vi "Check-client-activity.vi"(8 "error in (no error)":errorcluster, 9 "Check period":u32=5000 caption="Check period [ms]", 11 "ModComm in":T1) -> (0 "error out":errorcluster, 3 "ModComm out":T1)   [LabVIEW 2013, in "Server.lvlib" / "Server.lvclass"]
uses:
  Server.lvclass
  Object-reference.ctl
  Server.lvclass/Server.ctl
  Read Client IDs.vi
  Read Last contact.vi
  Read Heartbeat timeout.vi
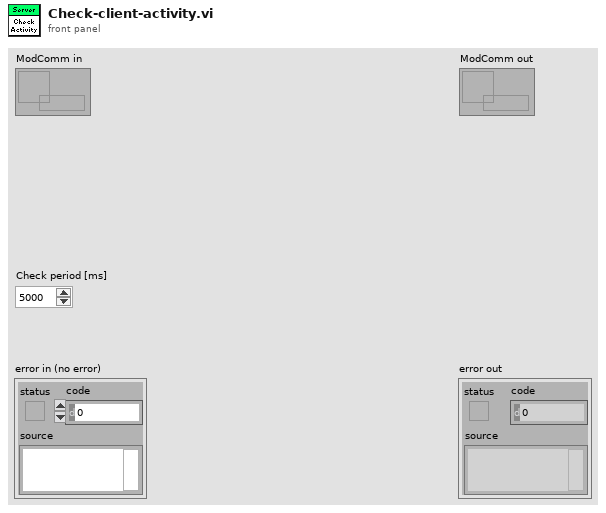
[diagram p1: front panel]
types:
  T1 = typedef "Server.lvlib/Server.lvclass/Object-reference.ctl" = refnum<data-value>
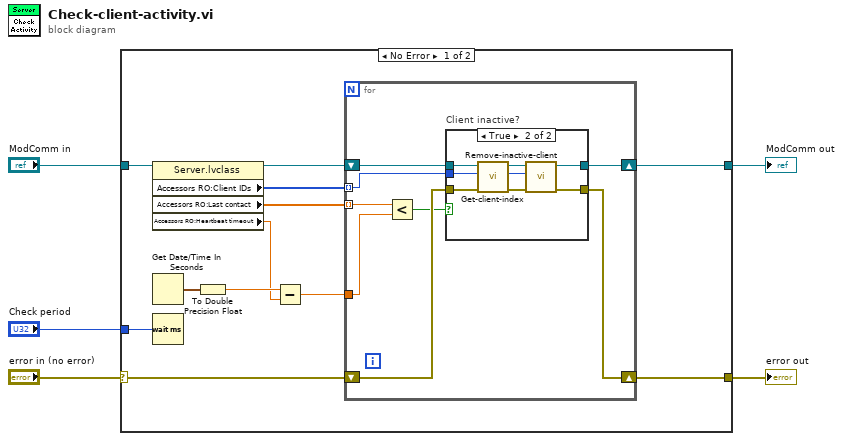
[diagram p0: block diagram]
diagram:
  n1 = case shown="No Error" "error in (no error)" {
    selector: "error in (no error)" -> [w7 w37]
    tunnel: [w6 w37] -> w4
    tunnel: [w8 w36] -> w2
    tunnel: "ModComm in" -> [w17 w36]
    tunnel: "Check period" -> [w16 _]
    frame No Error {
      n2 = property class="Server.lvclass"(reference=w17) -> (reference out=w9:T1, "Accessors RO:Client IDs"=w11:i32[], "Accessors RO:Last contact"=w12:dbl[], "Accessors RO:Heartbeat timeout"=w13:dbl)  [unwired: 1 in, 1 out]
      n3 = Get Date/Time In Seconds() -> (seconds since 1Jan1904=w15:timestamp)
      n4 = Wait (ms)(milliseconds to wait=w16) -> ()  [unwired: 1 out]
      n5 = To Double Precision Float(number=w15) -> (double precision float=w14:dbl)
      n6 = Subtract(x=w14, y=w13) -> (x-y=w10:dbl)
      n7 = for {
        tunnel: w12 -> [w25] mode=indexing
        tunnel: w11 -> [w18] mode=indexing
        tunnel: w10 -> [w24]
        shift-right: [w22] -> w8
        shift-left: w9 -> [w23]
        shift-right: [w20] -> w6
        shift-left: w7 -> [w21]
        n8 = Less?(x=w25, y=w24) -> (x < y?=w19:bool)
        n9 = case "Client inactive?" shown="True" w19 {
          tunnel: w23 -> [w27 w33]
          tunnel: [w27 w35] -> w22
          tunnel: w21 -> [w26 w29]
          tunnel: [w26 w34] -> w20
          tunnel: w18 -> [_ w30]
          frame False {
          }
          frame True {
            n10 = call "Get-client-index.vi"("error in (no error)"=w29, "Client ID"=w30, "ModComm in"=w33) -> ("error out"=w28:errorcluster, "Client index"=w31:i32, "ModComm out"=w32:T1)  [unwired: 6 in]
            n11 = call "Remove-inactive-client.vi"("error in (no error)"=w28, "Client index"=w31, "ModComm in"=w32) -> ("error out"=w34:errorcluster, "ModComm out"=w35:T1)  [unwired: 7 in]
          }
        }
      }
    }
    frame Error {
    }
  }
  "error out" <- w4
  "ModComm out" <- w2
